vi "Write Active Rectangle.vi"(8 "error in (no error)":errorcluster, 10 "Active Rectangle":refnum<class "Rectangle Settings.lvclass">, 11 "Setting Database in":refnum<class "Setting Database.lvclass">) -> (0 "error out":errorcluster, 3 "Setting Database out":refnum<class "Setting Database.lvclass">)   [LabVIEW 2019, in "Setting Database.lvclass"]
uses:
  Setting Database.lvclass
  Rectangle Settings/Rectangle Settings.lvclass
  Setting Database.lvclass/Setting Database.ctl
  ObjectSettings/Accessors/Read Enabled.vi
  ObjectSettings/Accessors/Write Enabled.vi
  C:/Users/Albro/Documents/GitHub/AFM-Lithography/lvsrc/Classes/Settings/ObjectSettings/ObjectSettings.lvclass
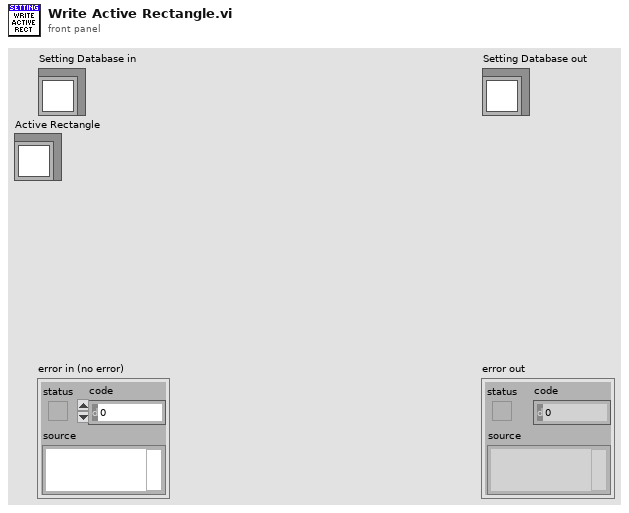
[diagram p1: front panel]
types:
  T1 = cluster{"Path":string, "Funnel":string, "Rectangle":string, "Dot":string}
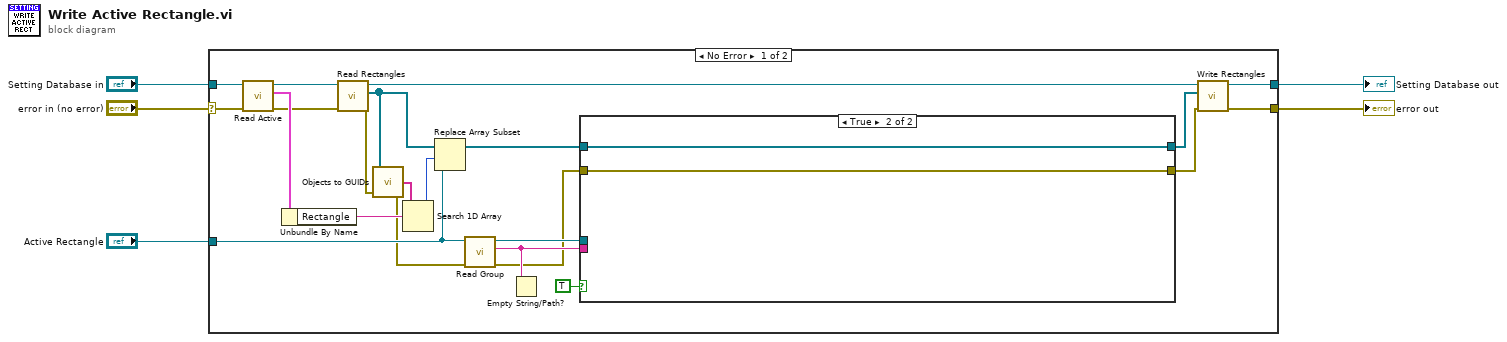
[diagram p0: block diagram]
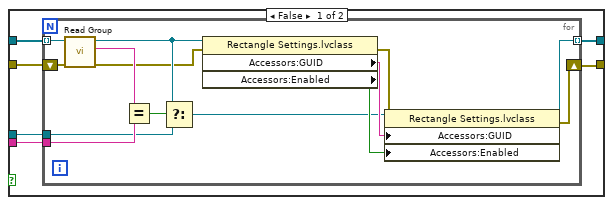
[diagram p2: hidden frame]
diagram:
  n1 = case shown="No Error" "error in (no error)" {
    selector: "error in (no error)" -> [w27 w51]
    tunnel: [w17 w51] -> w1
    tunnel: [w19 w50] -> w2
    tunnel: "Setting Database in" -> [w26 w50]
    tunnel: "Active Rectangle" -> [w24 _]
    frame No Error {
      n2 = call "Read Active.vi"("error in (no error)"=w27, "Setting Database in"=w26) -> ("error out"=w13:errorcluster, "Active"=w25:T1, "Setting Database out"=w15:refnum<class "Setting Database.lvclass">)  [unwired: 7 in]
      n3 = Unbundle By Name(w25) -> ("Rectangle"=w9:string)
      n4 = call "Read Rectangles.vi"("error in (no error)"=w13, "Setting Database in"=w15) -> ("error out"=w7:errorcluster, "Rectangles"=w11:refnum<class "Rectangle Settings.lvclass">[], "Setting Database out"=w14:refnum<class "Setting Database.lvclass">)  [unwired: 7 in]
      n5 = call "Objects to GUIDs.vi"("error in (no error)"=w7, "Objects"=w11) -> ("error out"=w6:errorcluster, "GUIDs"=w10:string[])  [unwired: 2 in]
      n6 = Search 1D Array(1D array=w10, element=w9) -> (index of element=w8:i32)  [unwired: 1 in]
      n7 = Replace Array Subset(array=w11, new element=w24, index=w8) -> (w23:refnum<class "Rectangle Settings.lvclass">[])
      n8 = call-dynamic "Read Group.vi"("error in (no error)"=w6, "ObjectSettings in"=w24) -> ("error out"=w20:errorcluster, "Group"=w22:string, "ObjectSettings out"=w21:refnum<class "Rectangle Settings.lvclass">)  [unwired: 7 in]
      n9 = Empty String/Path?(string/path=w22) -> ()  [unwired: 1 out]
      n10 = case shown="True" TRUE {
        tunnel: w23 -> [w32 w49]
        tunnel: [w30 w49] -> w16
        tunnel: w22 -> [w33 _]
        tunnel: w21 -> [w31 _]
        tunnel: w20 -> [w29 w48]
        tunnel: [w28 w48] -> w18
        frame False {
          n11 = for {
            tunnel: w33 -> [w45]
            tunnel: w32 -> [w47] mode=indexing
            tunnel: w31 -> [w44]
            tunnel: [w42] -> w30 mode=indexing
            shift-right: [w34] -> w28
            shift-left: w29 -> [w35]
            n12 = call-dynamic "Read Group.vi"("error in (no error)"=w35, "ObjectSettings in"=w47) -> ("error out"=w36:errorcluster, "Group"=w46:string, "ObjectSettings out"=w43:refnum<class "Rectangle Settings.lvclass">)  [unwired: 7 in]
            n13 = Equal?(x=w46, y=w45) -> (x = y?=w38:bool)
            n14 = Select(t=w43, s=w38, f=w44) -> (s? t:f=w39:refnum<class "Rectangle Settings.lvclass">)
            n15 = property class="Rectangle Settings.lvclass"(reference=w43, error in=w36) -> (error out=w37:errorcluster, "Accessors:GUID"=w41:string, "Accessors:Enabled"=w40:bool)  [unwired: 1 out]
            n16 = property class="Rectangle Settings.lvclass"(reference=w39, error in=w37, "Accessors:GUID"=w41, "Accessors:Enabled"=w40) -> (reference out=w42:refnum<class "Rectangle Settings.lvclass">, error out=w34:errorcluster)
          }
        }
        frame True {
        }
      }
      n17 = call "Write Rectangles.vi"("error in (no error)"=w18, "Rectangles"=w16, "Setting Database in"=w14) -> ("error out"=w17:errorcluster, "Setting Database out"=w19:refnum<class "Setting Database.lvclass">)  [unwired: 7 in]
    }
    frame Error {
    }
  }
  "error out" <- w1
  "Setting Database out" <- w2
